vi "output-save-header.vi"(3 "Image Details":T1={"image-laser-position"={"laser-x-position"=520, "laser-y-position"=696}, "magnification"=83.3333333} {"magnification" min=1.0 max=200.0 step=0.0001}, 4 "Spectrograph":T4={"Slit Width (µm)"=0.0, "Grating"=4, "Central Wavelength (nm)"=0.0, "Filter"=5, "Shutter"=0} {"Shutter" items=["Close", "Open"]; "Slit Width (µm)" min=10.0 max=2500.0 step=0.1 format="%.1f"; "Grating" items=["500 blz 300l/mm"=1, "1200 blz 300l/mm"=2, "1250 nm blaze"=3, "unknown"=4]; "Filter" items=["Empty"=5, "Longpass 900 nm"=4, "Longpass 715 nm"=3, "Longpass 475 nm"=2, "Longpass 320 nm"=1]; "Central Wavelength (nm)" min=200.0 max=2000.0 step=0.1 format="%.2f"}, 5 "PLE Excitation Input":T7, 6 "Detector":T3={"Current Detector"="CCD", "readout mode"=0, "Hbinning"=1, "Exposure Time"=0.2, "Cooling Read"={"iDus"=99, "Newton"=99, "Clara"=99}, "pre-amp"=9.0, "HSSpeed"=9.0} {"Exposure Time" format="%.3g"; "Hbinning" items=["1x"=1, "2x"=2, "4x"=4, "8x"=8, "16x"=16]; "readout mode" items=["Full Vertical Binning", "Image", "Vertical Binning"]}, 7 "background":T8={"BG shutter"=enum."with Open Shutter", "select background"=enum."skip"}, 8 "Lightsource":T2 {"Feedback Level" format="%.1f%"; "Power Level" format="%.1f%"; "Temperature (°C)" format="%.1f"}, 9 "Nanostage":T6={"x-axis"=150.0, "y-axis"=150.0, "z-axis"=150.0, "switch U/D"=TRUE, "switch L/R"=TRUE} {"y-axis" min=0.0 max=300.0 step=0.001 format="%.3f"; "x-axis" min=0.0 max=300.0 step=0.001 format="%.3f"; "z-axis" min=0.0 max=300.0 step=0.001 format="%.3f"}, 10 "Pixel Scaling":T5, 11 "general":T9={"Calibration Mode"=FALSE, "File Name"="File Name:", "User Name"="unknown", "Aborted?"=FALSE, "NKT System"=enum."SuperK Varia (VIS)"}) -> (1 "Header for .txt":string, 2 "Header for .ibw":string)   [LabVIEW 2017]
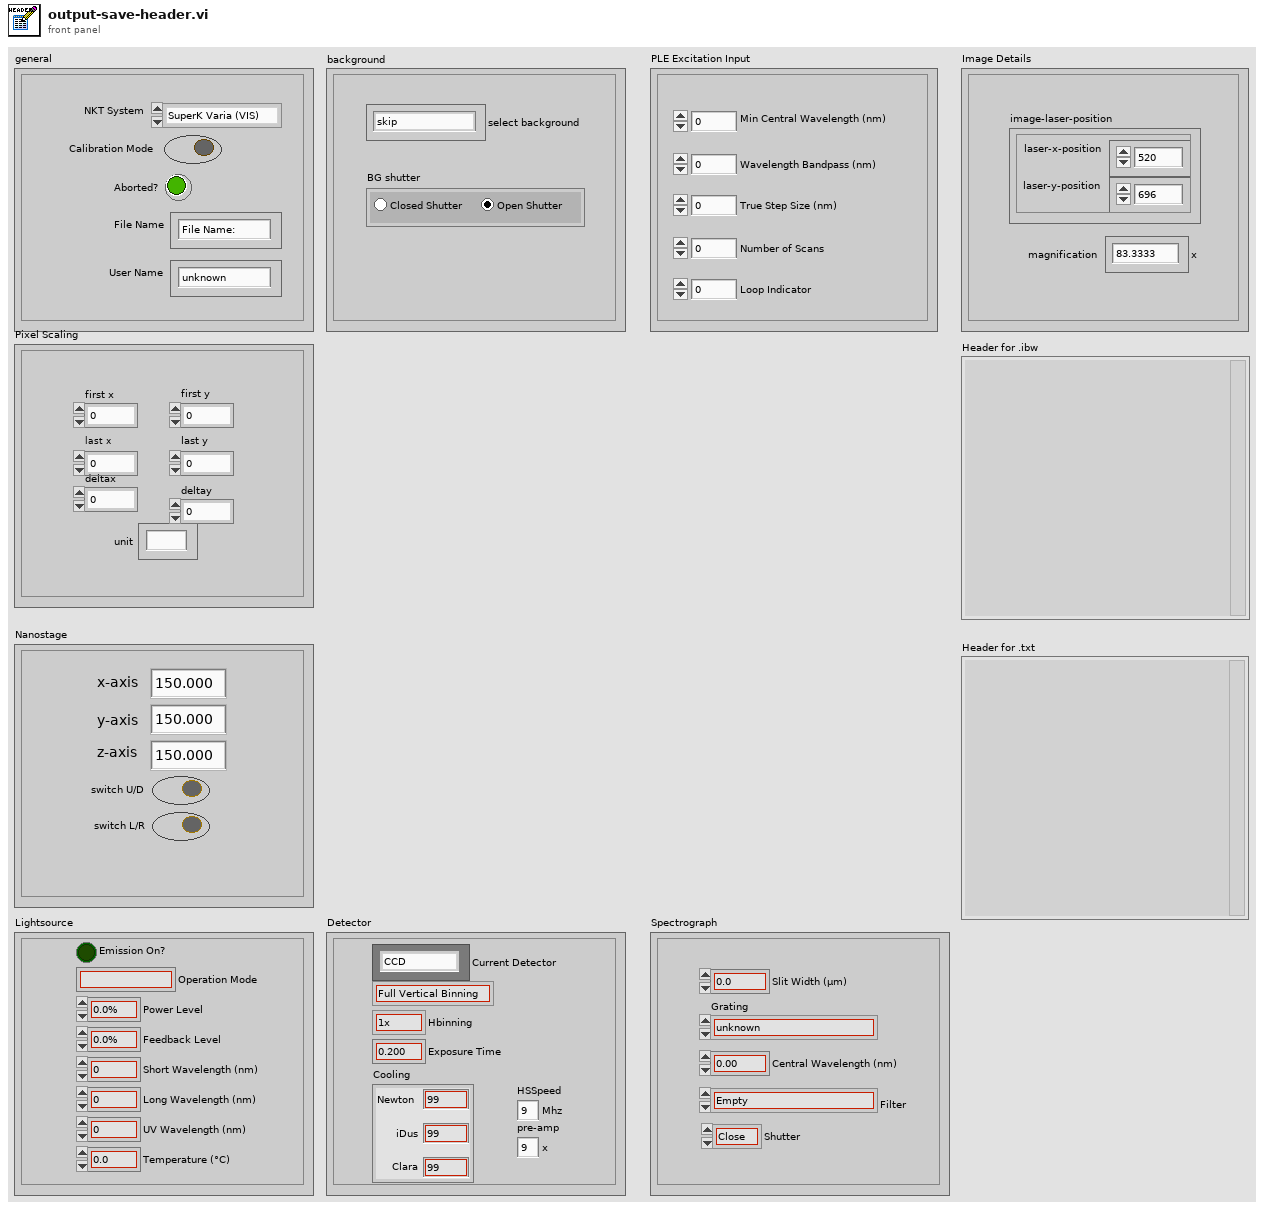
[diagram p1: front panel]
types:
  T1 = cluster{"image-laser-position":cluster{"laser-x-position":u16, "laser-y-position":u16}, "magnification":dbl}
  T2 = cluster{"Emission On?":bool, "Operation Mode":string, "Power Level":dbl, "Feedback Level":dbl, "Short Wavelength (nm)":i32, "Long Wavelength (nm)":i32, "UV Wavelength (nm)":i32, "Temperature (°C)":dbl}
  T3 = cluster{"Current Detector":string, "readout mode":u16, "Hbinning":u16, "Exposure Time":sgl, "Cooling Read":cluster{"iDus":i32, "Newton":i32, "Clara":i32}, "pre-amp":dbl, "HSSpeed":dbl}
  T4 = cluster{"Slit Width (µm)":dbl, "Grating":u16, "Central Wavelength (nm)":dbl, "Filter":u16, "Shutter":u16}
  T5 = cluster{"first x":sgl, "last x":sgl, "deltax":dbl, "first y":sgl, "last y":sgl, "deltay":dbl, "unit":string}
  T6 = cluster{"x-axis":dbl, "y-axis":dbl, "z-axis":dbl, "switch U/D":bool, "switch L/R":bool}
  T7 = cluster{"Min Central Wavelength (nm)":i32, "Wavelength Bandpass (nm)":i32, "True Step Size (nm) ":i32, "Number of Scans":i32, "Loop Indicator":i32}
  T8 = cluster{"BG shutter":enum32{"with Closed Shutter", "with Open Shutter"}, "select background":enum16{"skip", "single", "multiple"}}
  T9 = cluster{"Calibration Mode":bool, "File Name":string, "User Name":string, "Aborted?":bool, "NKT System":enum32{"SuperK Varia (VIS)", "Extend-UV"}}
  T10 = enum32{"with Closed Shutter", "with Open Shutter"}
  T11 = cluster{"laser-x-position":u16, "laser-y-position":u16}
  T12 = cluster{"laser-x-position":string, "laser-y-position":string}
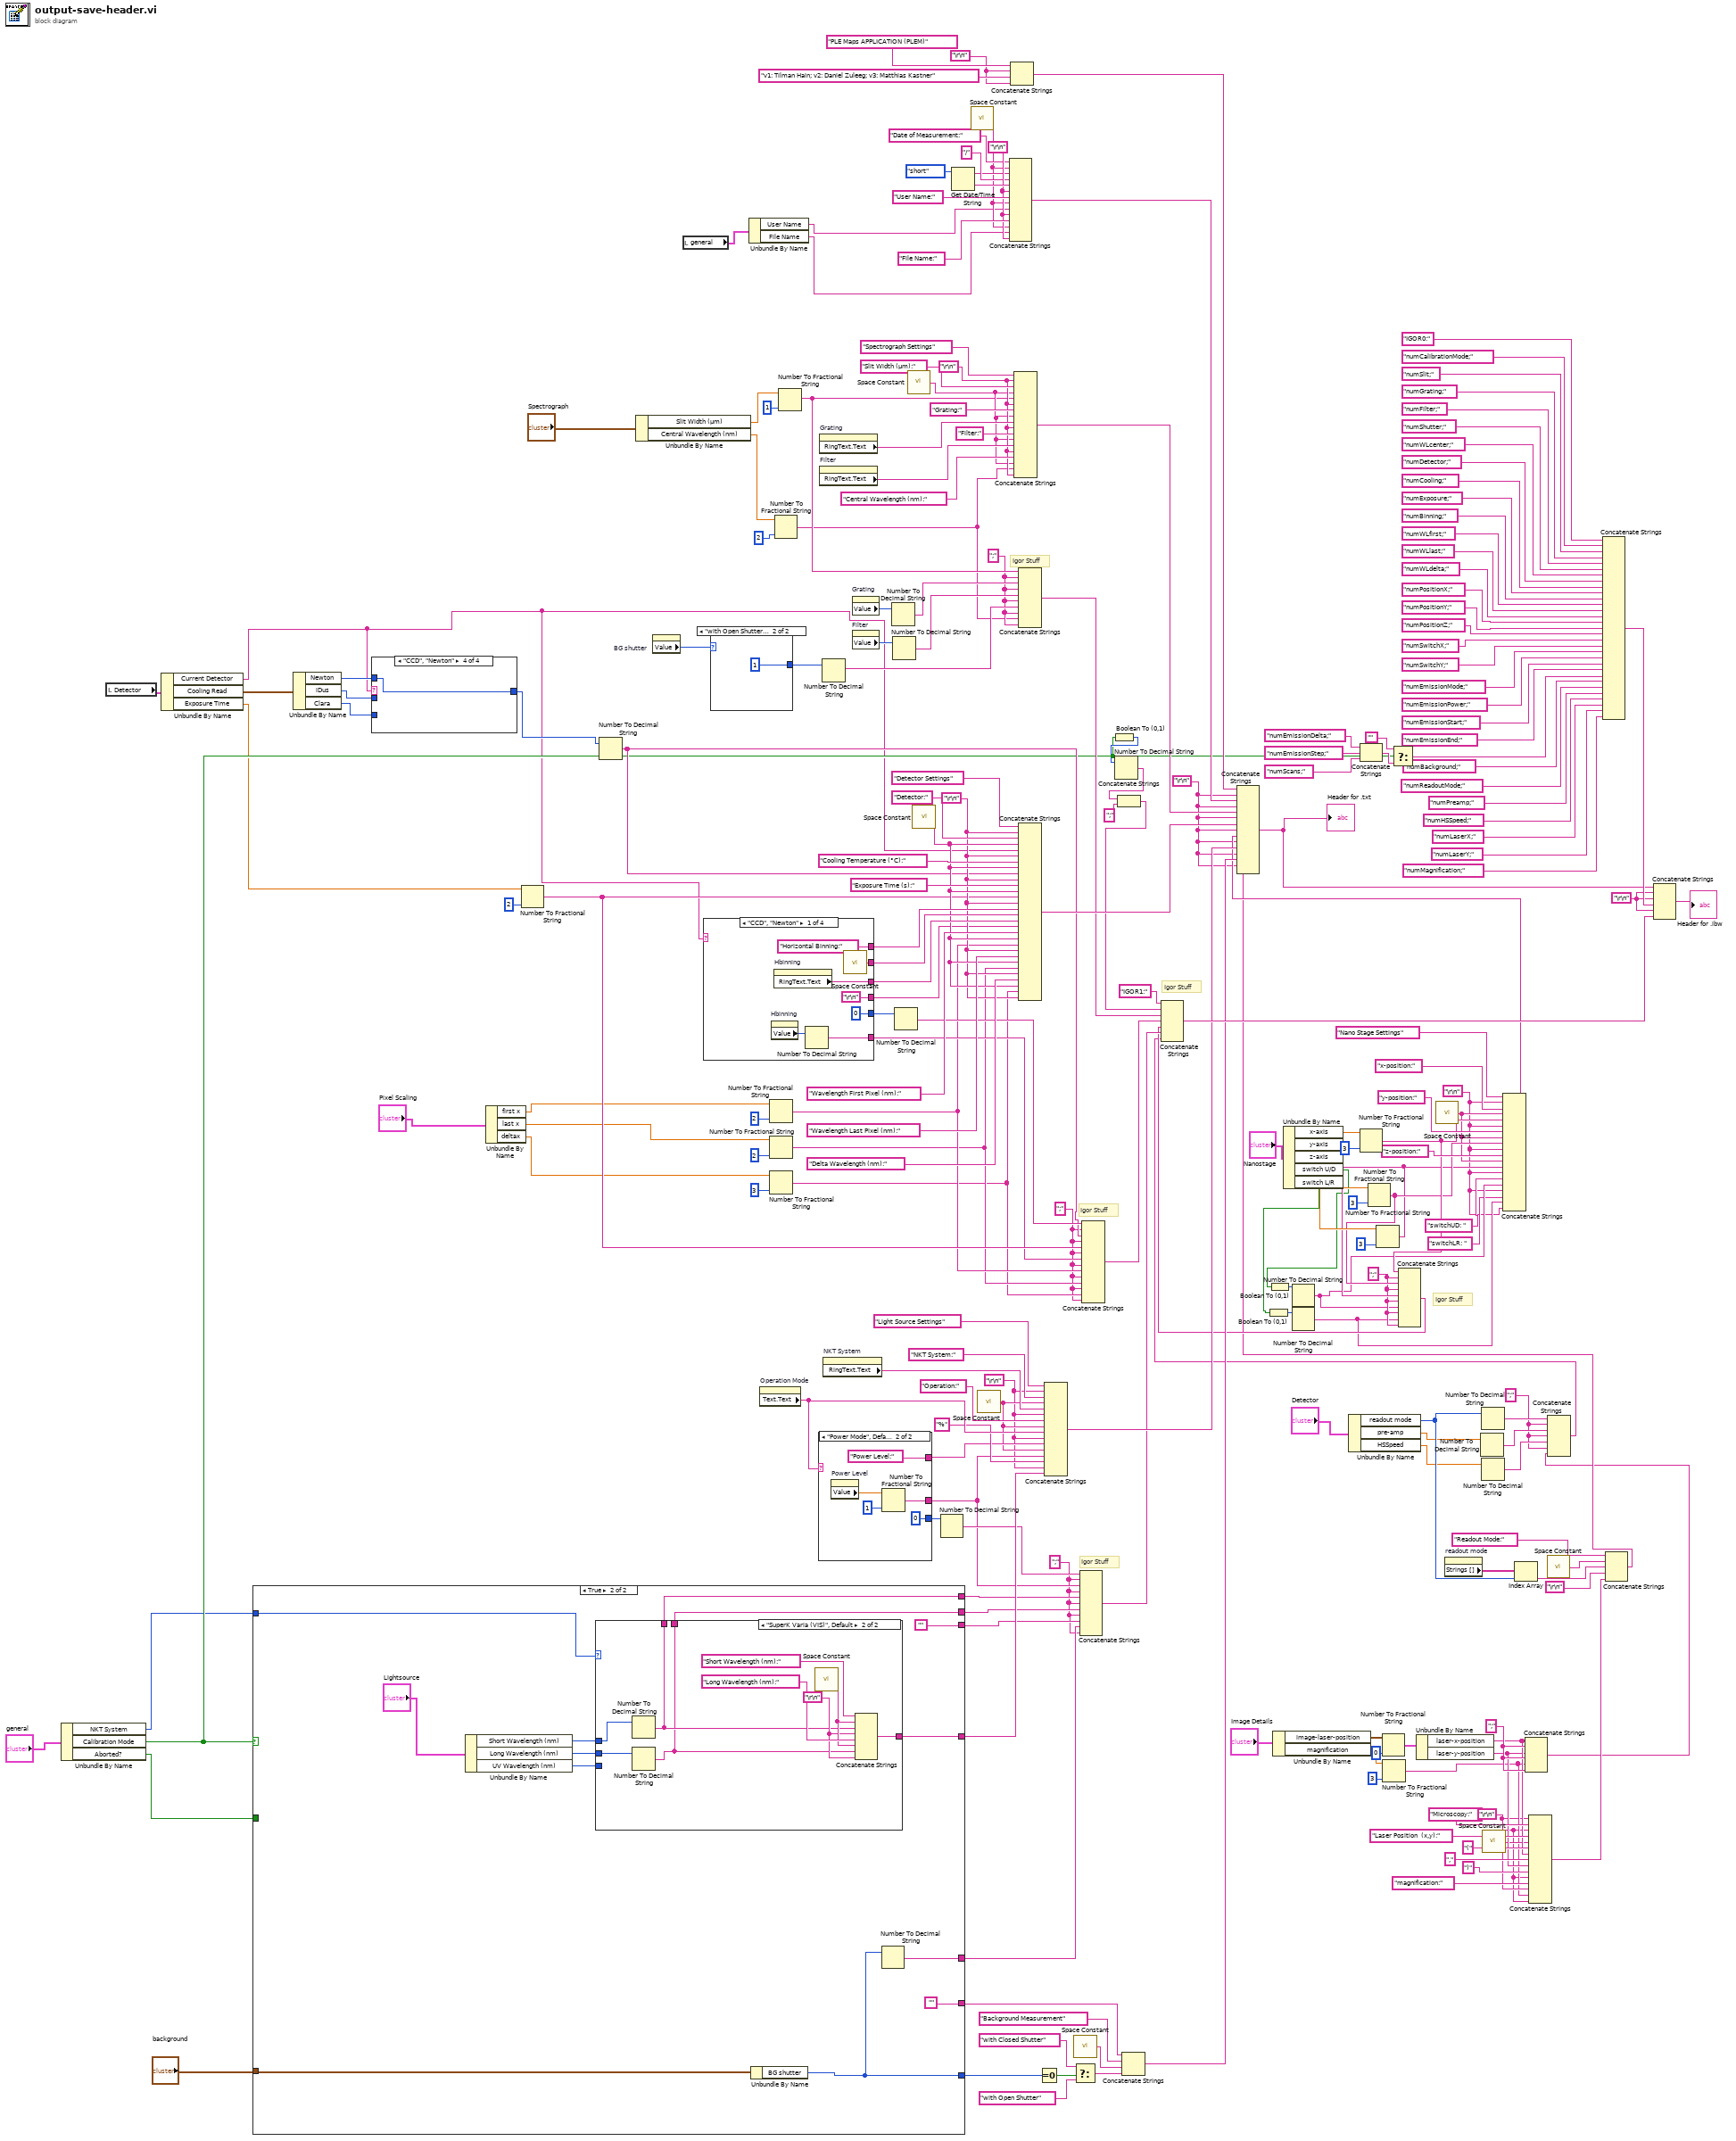
[diagram p0: block diagram]
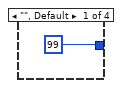
[diagram p2: hidden frame]
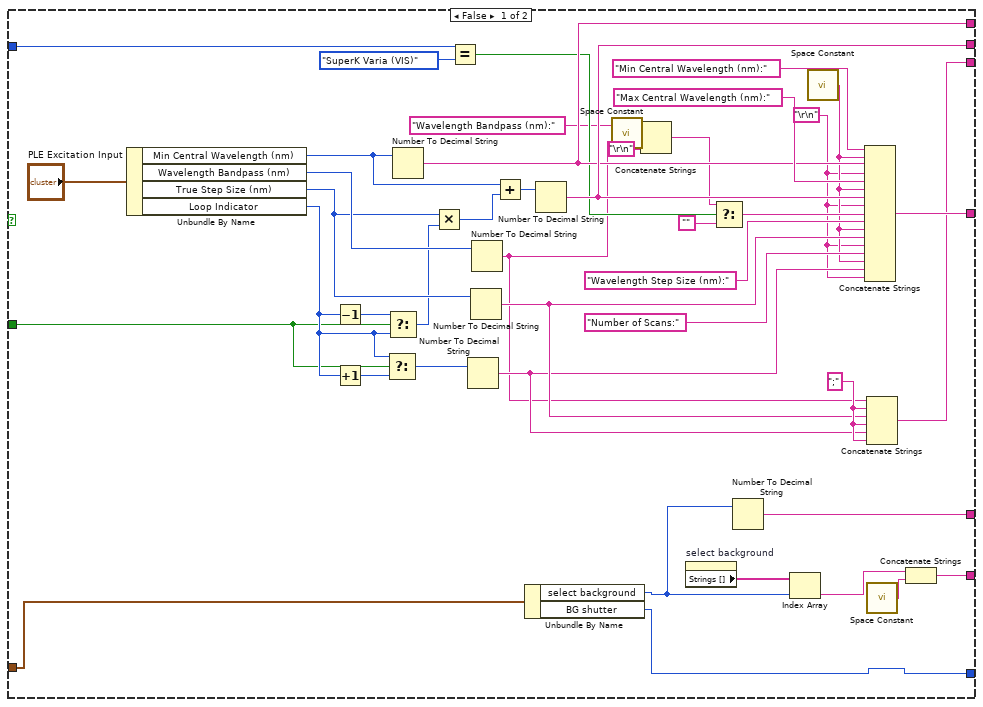
[diagram p5: hidden frame]
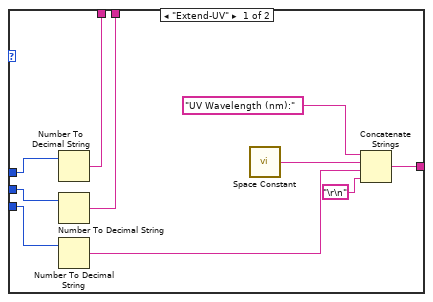
[diagram p6: hidden frame]
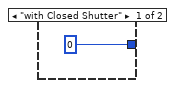
[diagram p7: hidden frame]
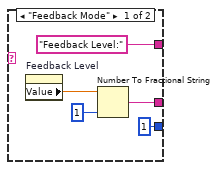
[diagram p8: hidden frame]
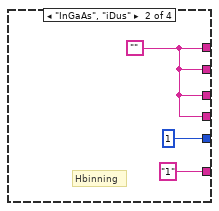
[diagram p9: hidden frame]
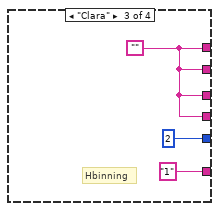
[diagram p10: hidden frame]
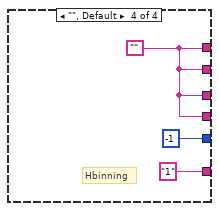
[diagram p11: hidden frame]
diagram:
  w19 = "\r\n"
  w35 = ";"
  w8 = ";"
  w41 = ";"
  w13 = "\r\n"
  w51 = ";"
  w129 = ";"
  w143 = "\r\n"
  w151 = ";"
  w186 = "\r\n"
  w75 = "\r\n"
  w108 = "\r\n"
  w192 = "\r\n"
  w217 = "\r\n"
  w209 = "\r\n"
  # "Igor Stuff"
  # "Igor Stuff"
  # "Igor Stuff"
  # "Igor Stuff"
  # "Igor Stuff"
  n1 = Unbundle By Name("general") -> ("NKT System"=w60:enum32{"SuperK Varia (VIS)", "Extend-UV"}, "Calibration Mode"=w68:bool, "Aborted?"=w64:bool)
  n2 = local read "Detector"() -> (w56:T3)
  n3 = Unbundle By Name(w56) -> ("Current Detector"=w54:string, "Cooling Read"=w55:cluster{"iDus":i32, "Newton":i32, "Clara":i32}, "Exposure Time"=w53:sgl)
  n4 = case shown="True" w68 {
    tunnel: [w261 w280] -> w175
    tunnel: [w255 ""] -> w139
    tunnel: [w229 w273] -> w138
    tunnel: [w254 w277] -> w124
    tunnel: [w253 w278] -> w125
    tunnel: [w251 ""] -> w118
    tunnel: [w250 w275] -> w117
    tunnel: w64 -> [w230 _]
    tunnel: w60 -> [w227 w271]
    tunnel: "background" -> [w228 w270]
    frame False {
      w252 = ";"
      w242 = "\r\n"
      n5 = Unbundle By Name("PLE Excitation Input") -> ("Min Central Wavelength (nm)"=w268:i32, "Wavelength Bandpass (nm)"=w264:i32, "True Step Size (nm)"=w263:i32, "Loop Indicator"=w257:i32)
      n6 = Decrement(x=w257) -> (x-1=w259:i32)
      n7 = Increment(x=w257) -> (x+1=w262:i32)
      n8 = Select(t=w257, s=w230, f=w262) -> (s? t:f=w260:i32)
      n9 = Select(t=w259, s=w230, f=w257) -> (s? t:f=w258:i32)
      n10 = Number To Decimal String(number=w268) -> (decimal integer string=w253:string)  [unwired: 1 in]
      n11 = Multiply(x=w263, y=w258) -> (x*y=w267:i32)
      n12 = Equal?(x=w227, y=enum32{"SuperK Varia (VIS)", "Extend-UV"}."SuperK Varia (VIS)" ("Select NKT System")) -> (x = y?=w240:bool)
      n13 = Number To Decimal String(number=w260) -> (decimal integer string=w243:string)  [unwired: 1 in]
      n14 = Number To Decimal String(number=w263) -> (decimal integer string=w246:string)  [unwired: 1 in]
      n15 = Number To Decimal String(number=w264) -> (decimal integer string=w238:string)  [unwired: 1 in]
      n16 = Add(x=w268, y=w267) -> (x+y=w266:i32)
      n17 = Unbundle By Name(w228) -> ("select background"=w231:enum16{"skip", "single", "multiple"}, "BG shutter"=w229:T10)
      n18 = Number To Decimal String(number=w266) -> (decimal integer string=w254:string)  [unwired: 1 in]
      n19 = call <vilib>:"Space Constant.vi"() -> ("String"=w237:string)
      n20 = Concatenate Strings("Wavelength Bandpass (nm):" ("string"), w237, w238, "\r\n") -> (w235:string)
      n21 = property on="select background" class="Enum (strict)"() -> ("Strings []"=w234:string[])  [unwired: 2 in, 2 out]
      n22 = Select(t=w235, s=w240, f="") -> (s? t:f=w248:string)
      n23 = Number To Decimal String(number=w231) -> (decimal integer string=w250:string)  [unwired: 1 in]
      n24 = Index Array(array=w234, index=w231) -> (element=w233:string)
      n25 = call <vilib>:"Space Constant.vi"() -> ("String"=w244:string)
      n26 = Concatenate Strings("Min Central Wavelength (nm):" ("string"), w244, w253, w242, "Max Central Wavelength (nm):" ("string"), w244, w254, w242, w248, "Wavelength Step Size (nm):" ("string"), w244, w246, w242, "Number of Scans:" ("string"), w244, w243, w242) -> (w261:string)
      n27 = Concatenate Strings(w238, w252, w246, w252, w243, w252) -> (w251:string)
      n28 = call <vilib>:"Space Constant.vi"() -> ("String"=w256:string)
      n29 = Concatenate Strings(w233, w256) -> (w255:string)
    }
    frame True {
      n30 = Unbundle By Name("Lightsource") -> ("Short Wavelength (nm)"=w282:i32, "Long Wavelength (nm)"=w281:i32, "UV Wavelength (nm)"=w274:i32)
      n31 = case shown="\"SuperK Varia (VIS)\", Default" w271 {
        tunnel: w282 -> [w292 w301]
        tunnel: w281 -> [w291 w300]
        tunnel: [w290 w295] -> w280
        tunnel: [w289 w294] -> w278
        tunnel: [w288 w293] -> w277
        tunnel: w274 -> [w287 _]
        frame "Extend-UV" {
          n32 = Number To Decimal String(number=w292) -> (decimal integer string=w289:string)  [unwired: 1 in]
          n33 = Number To Decimal String(number=w291) -> (decimal integer string=w288:string)  [unwired: 1 in]
          n34 = Number To Decimal String(number=w287) -> (decimal integer string=w284:string)  [unwired: 1 in]
          n35 = call <vilib>:"Space Constant.vi"() -> ("String"=w285:string)
          n36 = Concatenate Strings("UV Wavelength (nm):", w285, w284, "\r\n") -> (w290:string)
        }
        frame "SuperK Varia (VIS)", Default {
          w296 = "\r\n"
          n37 = Number To Decimal String(number=w301) -> (decimal integer string=w294:string)  [unwired: 1 in]
          n38 = Number To Decimal String(number=w300) -> (decimal integer string=w293:string)  [unwired: 1 in]
          n39 = call <vilib>:"Space Constant.vi"() -> ("String"=w297:string)
          n40 = Concatenate Strings("Short Wavelength (nm):", w297, w294, w296, "Long Wavelength (nm):", w297, w293, w296) -> (w295:string)
        }
      }
      n41 = Unbundle By Name(w270) -> ("BG shutter"=w273:T10)
      n42 = Number To Decimal String(number=w273) -> (decimal integer string=w275:string)  [unwired: 1 in]
    }
  }
  n43 = Unbundle By Name(w55) -> ("Newton"=w71:i32, "iDus"=w72:i32, "Clara"=w73:i32)
  n44 = case shown="\"CCD\", \"Newton\"" w54 {
    tunnel: w73 -> [_ _ w304 _]
    tunnel: w72 -> [_ w303 _ _]
    tunnel: w71 -> [_ _ _ w305]
    tunnel: [99 ("Clara") w303 w304 w305] -> w70
    frame "", Default {
    }
    frame "InGaAs", "iDus" {
    }
    frame "Clara" {
    }
    frame "CCD", "Newton" {
    }
  }
  n45 = Unbundle By Name("Pixel Scaling") -> ("first x"=w87:sgl, "last x"=w86:sgl, "deltax"=w85:dbl)
  n46 = Number To Fractional String(number=w53, precision (6)=i16 2) -> (F-format string=w134:string)  [unwired: 2 in]
  n47 = Number To Decimal String(number=w70) -> (decimal integer string=w135:string)  [unwired: 1 in]
  n48 = Unbundle By Name("Spectrograph") -> ("Slit Width (µm)"=w183:dbl, "Central Wavelength (nm)"=w170:dbl)
  n49 = property on="BG shutter" class="RadioBtnsControl (strict)"() -> ("Value"=w52:T10)  [unwired: 2 in, 2 out]
  n50 = local read "general"() -> (w67:T9)
  n51 = case shown="\"CCD\", \"Newton\"" w54 {
    tunnel: ["Horizontal Binning:" w315 w318 w321] -> w212
    tunnel: [w311 w315 w318 w321] -> w211
    tunnel: [w310 w315 w318 w321] -> w210
    tunnel: ["\r\n" w315 w318 w321] -> w177
    tunnel: [w307 "1" ("string") "1" ("string") "1" ("string")] -> w133
    tunnel: [0 1 2 -1] -> w137
    frame "CCD", "Newton" {
      n52 = property on="Hbinning" class="Ring (strict)"() -> ("Value"=w308:u16)  [unwired: 2 in, 2 out]
      n53 = property on="Hbinning" class="Ring (strict)"() -> ("RingText.Text"=w310:string)  [unwired: 2 in, 2 out]
      n54 = Number To Decimal String(number=w308) -> (decimal integer string=w307:string)  [unwired: 1 in]
      n55 = call <vilib>:"Space Constant.vi"() -> ("String"=w311:string)
    }
    frame "InGaAs", "iDus" {
      w315 = ""
      # "Hbinning"
    }
    frame "Clara" {
      w318 = ""
      # "Hbinning"
    }
    frame "", Default {
      w321 = ""
      # "Hbinning"
    }
  }
  n56 = case shown="\"with Open Shutter\", Default" w52 {
    tunnel: [0 1] -> w142
    frame "with Closed Shutter" {
    }
    frame "with Open Shutter", Default {
    }
  }
  n57 = Unbundle By Name(w67) -> ("User Name"=w65:string, "File Name"=w66:string)
  n58 = property on="Operation Mode" class="Str"() -> ("Text.Text"=w207:string)  [unwired: 2 in, 2 out]
  n59 = Number To Fractional String(number=w87, precision (6)=i16 2) -> (F-format string=w132:string)  [unwired: 2 in]
  n60 = Number To Fractional String(number=w86, precision (6)=i16 2) -> (F-format string=w131:string)  [unwired: 2 in]
  n61 = Number To Fractional String(number=w85, precision (6)=i16 3) -> (F-format string=w130:string)  [unwired: 2 in]
  n62 = Number To Fractional String(number=w170, precision (6)=i16 2) -> (F-format string=w150:string)  [unwired: 2 in]
  n63 = Number To Fractional String(number=w183, precision (6)=i16 1) -> (F-format string=w161:string)  [unwired: 2 in]
  n64 = case shown="\"Power Mode\", Default" w207 {
    tunnel: ["Feedback Level:" "Power Level:"] -> w205
    tunnel: [w325 w330] -> w126
    tunnel: [i16 1 ("width (-)") i16 0 ("width (-)")] -> w149
    frame "Feedback Mode" {
      n65 = property on="Feedback Level" class="DigNum (strict)"() -> ("Value"=w327:dbl)  [unwired: 2 in, 2 out]
      n66 = Number To Fractional String(number=w327, precision (6)=i16 1 ("width (-)")) -> (F-format string=w325:string)  [unwired: 2 in]
    }
    frame "Power Mode", Default {
      n67 = property on="Power Level" class="DigNum (strict)"() -> ("Value"=w331:dbl)  [unwired: 2 in, 2 out]
      n68 = Number To Fractional String(number=w331, precision (6)=i16 1 ("width (-)")) -> (F-format string=w330:string)  [unwired: 2 in]
    }
  }
  n69 = property on="Grating" class="Ring (strict)"() -> ("RingText.Text"=w222:string)  [unwired: 2 in, 2 out]
  n70 = property on="Filter" class="Ring (strict)"() -> ("RingText.Text"=w220:string)  [unwired: 2 in, 2 out]
  n71 = Number To Decimal String(number=w142) -> (decimal integer string=w156:string)  [unwired: 1 in]
  n72 = property on="NKT System" class="Enum (strict)"() -> ("RingText.Text"=w111:string)  [unwired: 2 in, 2 out]
  n73 = property on="Grating" class="Ring (strict)"() -> ("Value"=w160:u16)  [unwired: 2 in, 2 out]
  n74 = property on="Filter" class="Ring (strict)"() -> ("Value"=w158:u16)  [unwired: 2 in, 2 out]
  n75 = Number To Decimal String(number=w160) -> (decimal integer string=w159:string)  [unwired: 1 in]
  n76 = Number To Decimal String(number=w158) -> (decimal integer string=w157:string)  [unwired: 1 in]
  n77 = Number To Decimal String(number=w137) -> (decimal integer string=w136:string)  [unwired: 1 in]
  n78 = call <vilib>:"Space Constant.vi"() -> ("String"=w202:string)
  n79 = call <vilib>:"Space Constant.vi"() -> ("String"=w193:string)
  n80 = Number To Decimal String(number=w149) -> (decimal integer string=w127:string)  [unwired: 1 in]
  n81 = Get Date/Time String(date format (0)=enum16{"short", "long", "abbreviated"}."short") -> (date string=w173:string, time string=w189:string)  [unwired: 2 in]
  n82 = call <vilib>:"Space Constant.vi"() -> ("String"=w171:string)
  n83 = call <vilib>:"Space Constant.vi"() -> ("String"=w110:string)
  n84 = Concatenate Strings("Date of Measurement:", w171, w173, "/" ("string"), w189, w186, "User Name:", w171, w65, w186, "File Name:", w171, w66, w186) -> (w185:string)
  n85 = Concatenate Strings("PLE Maps APPLICATION (PLEM)" ("string"), w209, "v1: Tilman Hain; v2: Daniel Zuleeg; v3: Matthias Kastner" ("string"), w209) -> (w190:string)
  n86 = Concatenate Strings("Spectrograph Settings" ("string"), w217, "Slit Width (µm):" ("string"), w202, w161, w217, "Grating:" ("string"), w202, w222, w217, "Filter:" ("string"), w202, w220, w217, "Central Wavelength (nm):" ("string"), w202, w150, w217) -> (w203:string)
  n87 = Concatenate Strings(w161, w151, w159, w151, w157, w151, w156, w151, w150, w151) -> (w147:string)
  n88 = Concatenate Strings("Detector Settings" ("string"), w192, "Detector:" ("string"), w193, w54, w192, "Cooling Temperature (°C):" ("string"), w193, w135, w192, "Exposure Time (s):" ("string"), w193, w134, w192, w212, w211, w210, w177, "Wavelength First Pixel (nm):", w193, w132, w192, "Wavelength Last Pixel (nm):", w193, w131, w192, "Delta Wavelength (nm):", w193, w130, w192) -> (w204:string)
  n89 = Equal To 0?(x=w138) -> (x = 0?=w201:bool)
  n90 = Concatenate Strings("Light Source Settings" ("string"), w108, "NKT System:" ("string"), w110, w111, w108, "Operation:" ("string"), w110, w207, w108, w205, w110, w126, "%", w108, w175) -> (w105:string)
  n91 = call <vilib>:"Space Constant.vi"() -> ("String"=w176:string)
  n92 = Select(t="with Closed Shutter", s=w201, f="with Open Shutter") -> (s? t:f=w197:string)
  n93 = Concatenate Strings(w127, w51, w126, w51, w125, w51, w124, w51, w118, w117, w51) -> (w92:string)
  n94 = Concatenate Strings(w136, w129, w135, w129, w134, w129, w133, w129, w132, w129, w131, w129, w130, w129) -> (w128:string)
  n95 = Boolean To (0,1)(Boolean=w68) -> (0, 1=w115:i16)
  n96 = Number To Decimal String(number=w115) -> (decimal integer string=w114:string)  [unwired: 1 in]
  n97 = Concatenate Strings(w114, ";") -> (w112:string)
  n98 = Concatenate Strings(w139, "Background Measurement", w176, w197) -> (w106:string)
  n99 = Unbundle By Name("Image Details") -> ("image-laser-position"=w31:T11, "magnification"=w33:dbl)
  n100 = Unbundle By Name("Nanostage") -> ("x-axis"=w99:dbl, "y-axis"=w98:dbl, "z-axis"=w97:dbl, "switch U/D"=w38:bool, "switch L/R"=w37:bool)
  n101 = Boolean To (0,1)(Boolean=w37) -> (0, 1=w39:i16)
  n102 = Boolean To (0,1)(Boolean=w38) -> (0, 1=w40:i16)
  n103 = Number To Decimal String(number=w40) -> (decimal integer string=w16:string)  [unwired: 1 in]
  n104 = Number To Decimal String(number=w39) -> (decimal integer string=w14:string)  [unwired: 1 in]
  n105 = Unbundle By Name("Detector") -> ("readout mode"=w57:u16, "pre-amp"=w12:dbl, "HSSpeed"=w11:dbl)
  n106 = Concatenate Strings("numEmissionDelta;", "numEmissionStep;", "numScans;") -> (w119:string)
  n107 = Number To Fractional String(number=w99, precision (6)=i16 3) -> (F-format string=w95:string)  [unwired: 2 in]
  n108 = Number To Fractional String(number=w98, precision (6)=i16 3) -> (F-format string=w94:string)  [unwired: 2 in]
  n109 = Number To Fractional String(number=w97, precision (6)=i16 3) -> (F-format string=w93:string)  [unwired: 2 in]
  n110 = Number To Fractional String(number=w31, precision (6)=i16 0) -> (F-format string=w30:T12)  [unwired: 2 in]
  n111 = Number To Fractional String(number=w33, precision (6)=i16 3) -> (F-format string=w20:string)  [unwired: 2 in]
  n112 = Select(t="", s=w68, f=w119) -> (s? t:f=w48:string)
  n113 = Concatenate Strings(w95, w41, w94, w41, w93, w41, w16, w41, w14, w41) -> (w91:string)
  n114 = Unbundle By Name(w30) -> ("laser-x-position"=w24:string, "laser-y-position"=w23:string)
  n115 = call <vilib>:"Space Constant.vi"() -> ("String"=w36:string)
  n116 = property on="readout mode" class="Ring (strict)"() -> ("Strings []"=w80:string[])  [unwired: 2 in, 2 out]
  n117 = Number To Decimal String(number=w12) -> (decimal integer string=w10:string)  [unwired: 1 in]
  n118 = Number To Decimal String(number=w57) -> (decimal integer string=w82:string)  [unwired: 1 in]
  n119 = Number To Decimal String(number=w11) -> (decimal integer string=w9:string)  [unwired: 1 in]
  n120 = call <vilib>:"Space Constant.vi"() -> ("String"=w21:string)
  n121 = Concatenate Strings("Nano Stage Settings" ("string"), w13, "x-position:" ("string"), w36, w95, w13, "y-position:" ("string"), w36, w94, w13, "z-position:" ("string"), w36, w93, w13, "switchUD: " ("string"), w16, w13, "switchLR: " ("string"), w14, w13) -> (w96:string)
  n122 = Index Array(array=w80, index=w57) -> (element=w78:string)
  n123 = Concatenate Strings(w24, w35, w23, w35, w20, w35) -> (w7:string)
  n124 = Concatenate Strings(w19, "Microscopy:" ("string"), w19, "Laser Position  (x,y):" ("string"), w21, "(" ("string"), w24, "," ("string"), w23, ")" ("string"), w19, "magnification:" ("string"), w21, w20, w19) -> (w18:string)
  n125 = call <vilib>:"Space Constant.vi"() -> ("String"=w77:string)
  n126 = Concatenate Strings(w82, w8, w10, w8, w9, w8, w7) -> (w81:string)
  n127 = Concatenate Strings("IGOR1:", w112, w147, w128, w91, w92, w81) -> (w146:string)
  n128 = Concatenate Strings("IGOR0:", "numCalibrationMode;", "numSlit;", "numGrating;", "numFilter;", "numShutter;", "numWLcenter;", "numDetector;", "numCooling;", "numExposure;", "numBinning;", "numWLfirst;", "numWLlast;", "numWLdelta;", "numPositionX;", "numPositionY;", "numPositionZ;", "numSwitchX;", "numSwitchY;", "numEmissionMode;", "numEmissionPower;", "numEmissionStart;", "numEmissionEnd;", w48, "numBackground;", "numReadoutMode;" ("string"), "numPreamp;" ("string"), "numHSSpeed;" ("string"), "numLaserX;" ("string"), "numLaserY;" ("string"), "numMagnification;" ("string")) -> (w148:string)
  n129 = Concatenate Strings("Readout Mode:" ("string"), w77, w78, "\r\n", w18) -> (w74:string)
  n130 = Concatenate Strings(w190, w75, w185, w75, w203, w75, w204, w75, w96, w75, w105, w75, w106, w75, w74) -> (w144:string)
  "Header for .txt" <- w144
  n131 = Concatenate Strings(w144, w143, w143, w148, w143, w146) -> (→"Header for .ibw":string)
